vi "Create Size.vi"(8 "error in (no error)":errorcluster caption="错误输入（无错误）", 10 "Height":dbl, 11 "Width":dbl) -> (0 "error out":errorcluster caption="错误输出", 3 "Size 输出":refnum<class "Size.lvclass"> caption="DNL_LabVIEW Object out")   [LabVIEW 2011, in "Size.lvclass"]
uses:
  Size.lvclass
panel:
  in  "Size 输入":refnum<class "Size.lvclass"> caption="DNL_LabVIEW Object in"
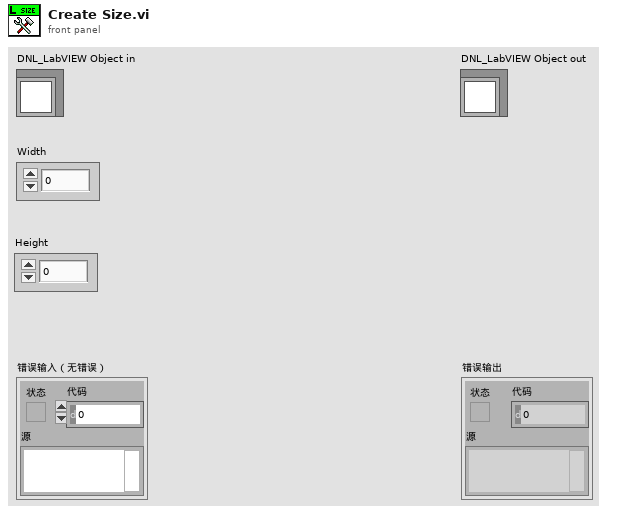
[diagram p1: front panel]
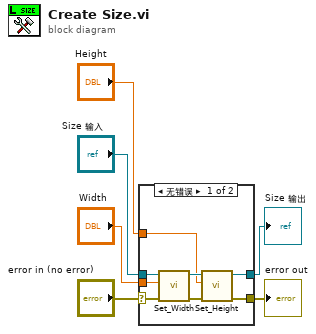
[diagram p0: block diagram]
diagram:
  n1 = case shown="无错误" "error in (no error)" {
    selector: "error in (no error)" -> [w12 w16]
    tunnel: [w7 w16] -> w5
    tunnel: [w8 w15] -> w3
    tunnel: "Size 输入" -> [w13 w15]
    tunnel: "Width" -> [w14 _]
    tunnel: "Height" -> [w10 _]
    frame No Error {
      n2 = call "Set_Width.vi"("error in (no error)"=w12, "Width"=w14, "Size输入"=w13) -> ("error out"=w9:errorcluster, "Size输出"=w11:refnum<class "Size.lvclass">)  [unwired: 7 in]
      n3 = call "Set_Height.vi"("error in (no error)"=w9, "Height"=w10, "Size输入"=w11) -> ("error out"=w7:errorcluster, "Size输出"=w8:refnum<class "Size.lvclass">)  [unwired: 7 in]
    }
    frame Error {
    }
  }
  "error out" <- w5
  "Size 输出" <- w3
